vi "PNA_Parse_Time-Date.vi"(8 "error in (no error)":errorcluster, 10 "SYST:DATE (IN)":string, 11 "SYST:TIME (IN)":string) -> (0 "error out":errorcluster, 1 "Time/Date Out (Str)":string, 2 "Time Stamp":timestamp, 3 "Date Out (str)":string, 5 "Time Out (str)":string)   [LabVIEW 2018]
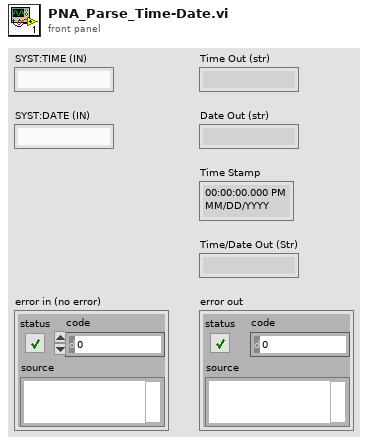
[diagram p1: front panel]
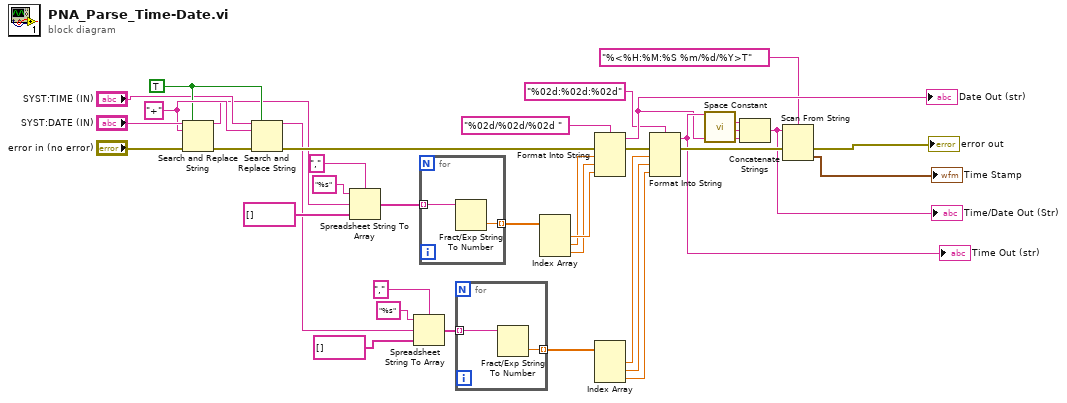
[diagram p0: block diagram]
diagram:
  w11 = TRUE ("replace all? (F)")
  w12 = "+" ("search string")
  n1 = Search and Replace String(replace all?=w11, input string="SYST:DATE (IN)", search string=w12, error in="error in (no error)") -> (result string=w2:string, error out=w1:errorcluster)  [unwired: 4 in, 2 out]
  n2 = Search and Replace String(replace all?=w11, input string="SYST:TIME (IN)", search string=w12, error in=w1) -> (result string=w3:string, error out=w34:errorcluster)  [unwired: 4 in, 2 out]
  n3 = Spreadsheet String To Array(delimiter (Tab)=",", format string="%s", spreadsheet string=w2, array type (2D Dbl)=string[] [] ("array")) -> (array=w16:string[])
  n4 = Spreadsheet String To Array(delimiter (Tab)=",", format string="%s", spreadsheet string=w3, array type (2D Dbl)=string[] [] ("array")) -> (array=w15:string[])
  n5 = for {
    tunnel: w16 -> [w38] mode=indexing
    tunnel: [w37] -> w17 mode=indexing
    n6 = Fract/Exp String To Number(string=w38) -> (number=w37:dbl)  [unwired: 3 in, 1 out]
  }
  n7 = for {
    tunnel: w15 -> [w40] mode=indexing
    tunnel: [w39] -> w22 mode=indexing
    n8 = Fract/Exp String To Number(string=w40) -> (number=w39:dbl)  [unwired: 3 in, 1 out]
  }
  n9 = Index Array(array=w17) -> (element #1=w20:dbl, element #2=w18:dbl, element #3=w19:dbl)  [unwired: 3 in]
  n10 = Format Into String(format string="%02d/%02d/%02d " ("initial string"), error in=w34, w18, w19, w20) -> (resulting string=w30:string, error out=w35:errorcluster)  [unwired: 1 in]
  "Date Out (str)" <- w30
  n11 = Index Array(array=w22) -> (element #1=w23:dbl, element #2=w24:dbl, element #3=w25:dbl)  [unwired: 3 in]
  n12 = Format Into String(format string="%02d:%02d:%02d" ("initial string"), error in=w35, w23, w24, w25) -> (resulting string=w31:string, error out=w36:errorcluster)  [unwired: 1 in]
  "Time Out (str)" <- w31
  n13 = call <vilib>:"Space Constant.vi"() -> ("String"=w33:string)
  n14 = Concatenate Strings(w31, w33, w30) -> (w32:string)
  "Time/Date Out (Str)" <- w32
  n15 = Scan From String(format string="%<%H:%M:%S %m/%d/%Y>T", input string=w32, error in=w36) -> (error out=→"error out":errorcluster, output 1=→"Time Stamp":timestamp)  [unwired: 2 in, 2 out]
